vi "AdressRead.vi"(0 "LINX Resource in":T1, 2 "I2C Slave Address":u8, 3 "Adress":u8[](array[numeric])=[243] format="%x", 5 "error in (no error)":errorcluster, 8 "I2C Channel":u8, 10 "milliseconds to wait":u32) -> (14 "LINX Resource out":T1, 17 "Data":u8[](array[numeric]), 19 "error out":errorcluster)   [LabVIEW 2014, in "BME280.lvclass"]
uses:
  BME280.lvclass
  <vilib>/MakerHub/LINX/Private/Type Defs/LINX Ref.ctl
  <vilib>/MakerHub/LINX/Private/Type Defs/Platform.ctl
  <vilib>/MakerHub/LINX/Private/Type Defs/Interface.ctl
  <vilib>/MakerHub/LINX/Private/Device/Type Defs/LINX Device Config.ctl
  <vilib>/MakerHub/LINX/Private/Device/Type Defs/TCP Config.ctl
  <vilib>/MakerHub/LINX/Private/Device/Type Defs/Channels.ctl
  <vilib>/MakerHub/LINX/Private/Local IO/LinxI2cWrite.vi
  <vilib>/MakerHub/LINX/Public/Utilities/Check Channel.vi
  <vilib>/MakerHub/LINX/Private/Local IO/Handle Errors.vi
  <vilib>/MakerHub/LINX/Private/Utilties/Generate Error.vi
  <vilib>/MakerHub/LINX/LMH-LINX.lvlib
  <vilib>/MakerHub/LINX/Private/Device/Device.lvlib
panel:
  out "size(s)":i32
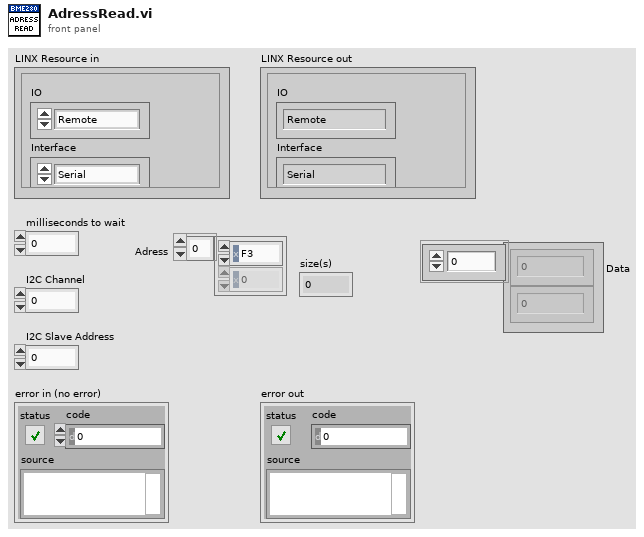
[diagram p1: front panel]
types:
  T1 = typedef "LMH-LINX.lvlib/LINX Ref.ctl" = cluster{"IO":T2, "Interface":T3, "LINX Device Config":T4}
  T2 = typedef "LMH-LINX.lvlib/Platform.ctl" = enum16{"Remote", "Local"}
  T3 = typedef "LMH-LINX.lvlib/Interface.ctl" = enum16{"Serial", "TCP"}
  T4 = typedef "LMH-LINX.lvlib/Device.lvlib/LINX Device Config.ctl" = cluster{"Interface":T3, "COM Port":refnum<visa-resource-name>, "TCP Configuration":T5, "Device Family":u8, "Device ID":u8, "Device Name":string, "TCP Ref":refnum<k5>, "Channels":T6}
  T5 = typedef "LMH-LINX.lvlib/Device.lvlib/TCP Config.ctl" = cluster{"IP Address":string, "Port":u16}
  T6 = typedef "LMH-LINX.lvlib/Channels.ctl" = cluster{"DI":u8[], "DO":u8[], "AI":u8[], "AO":u8[], "PWM":u8[], "QE":u8[], "UART":u8[], "I2C 2":u8[], "SPI":u8[], "CAN":u8[], "Servo":u8[], "AI Ref (V)":dbl, "AI Resolution (Bits)":u8, "AO Ref (V)":dbl, "AO Resolution (Bits)":u8}
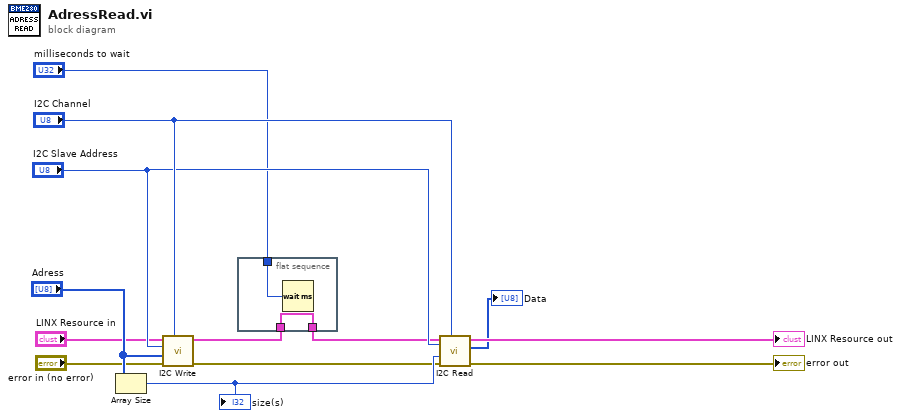
[diagram p0: block diagram]
diagram:
  n1 = Array Size(array="Adress") -> (size(s)=w12:i32)
  "size(s)" <- w12
  n2 = call <vilib>:"I2C Write.vi"("I2C Channel"="I2C Channel", "Error In"="error in (no error)", "Data"="Adress", "I2C Slave Address (0)"="I2C Slave Address", "LINX Resource"="LINX Resource in") -> ("Error Out"=w3:errorcluster, "LINX Resource"=w5:T1)  [unwired: 5 in]
  n3 = flat-sequence {
    tunnel: [w15] -> w6
    tunnel: w5 -> [w15]
    tunnel: "milliseconds to wait" -> [w14]
    frame #0 {
      n4 = Wait (ms)(milliseconds to wait=w14) -> ()  [unwired: 1 out]
    }
  }
  n5 = call <vilib>:"I2C Read.vi"("I2C Channel"="I2C Channel", "Error In"=w3, "Bytes To Read"=w12, "I2C Slave Address (0)"="I2C Slave Address", "LINX Resource"=w6) -> ("Error Out"=→"error out":errorcluster, "Data"=→"Data":u8[], "LINX Resource"=→"LINX Resource out":T1)  [unwired: 4 in]
